vi "_PC_Pub lockPrompt.vi"(0 "Enable":bool=TRUE, 5 "error in (no error)":errorcluster) -> (17 "New Group Name":string, 18 "OK":bool, 19 "error out":errorcluster)   [LabVIEW 2018]
doc: "Displays a standard dialog box that prompts users to enter information, such as a user name and password.\n--------------------\n\nThis Express VI is configured as follows:\n\nMessage to Display to the User:Add Group Name?\nThe inputs are: \nText Entry Box: New Group Name"
panel:
  in  "New Group Name":string
  out "String":string="Add Group Name?"
  in  "Cancel":bool
  in  "OK2":bool
  in  "OK1":bool
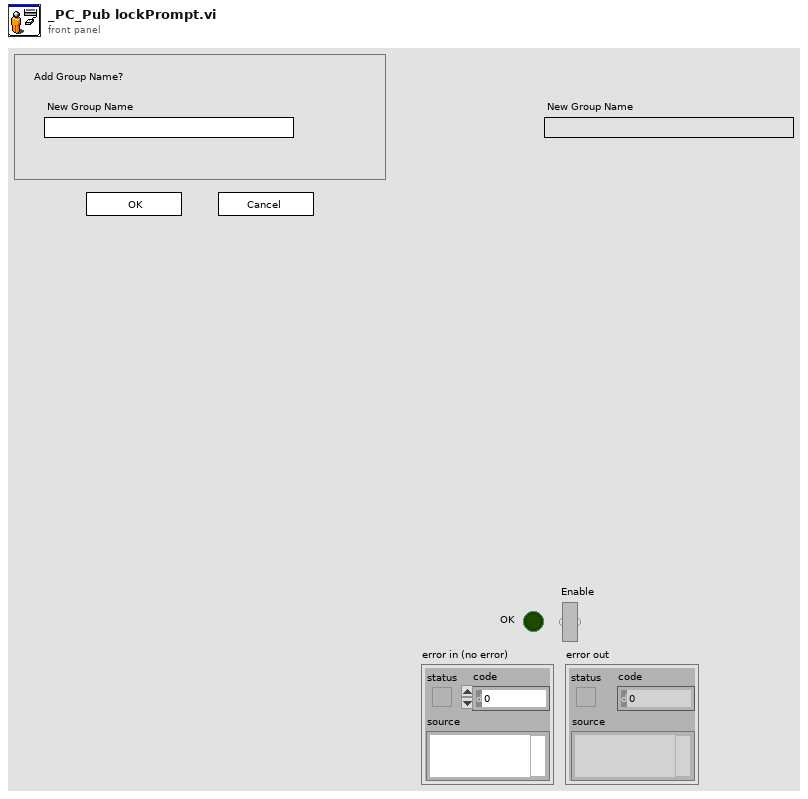
[diagram p1: front panel]
types:
  T1 = cluster{"Input Name":string, "Input Data Type":i32}[]
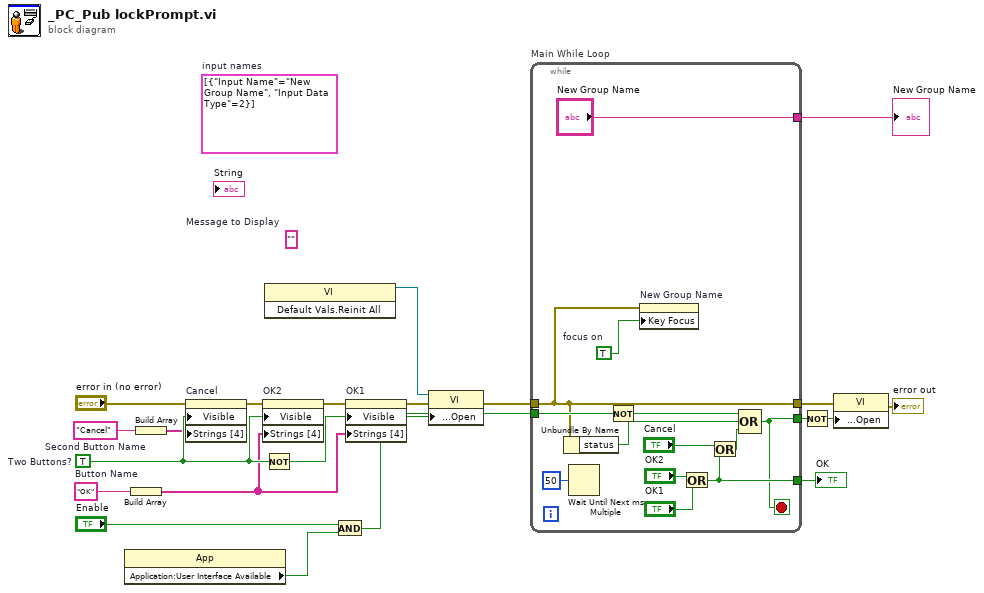
[diagram p0: block diagram]
diagram:
  (unwired) T1 [{"Input Name"="New Group Name", "Input Data Type"=2}]  # input names
  w13 = "Cancel"  # Second Button Name
  w11 = "OK"  # Button Name
  (unwired) ""  # Message to Display
  w21 = TRUE  # Two Buttons?
  n1 = property class="App"() -> ("Application:User Interface Available"=w3:bool)  [unwired: 2 in, 2 out]
  n2 = Build Array(w11) -> (w12:string[])
  n3 = Build Array(w13) -> (w14:string[])
  n4 = property on="Cancel" class="Bool"(error in="error in (no error)", "Visible"=w21, "Strings [4]"=w14) -> (error out=w18:errorcluster)  [unwired: 1 in, 1 out]
  n5 = property on="OK2" class="Bool"(error in=w18, "Visible"=w21, "Strings [4]"=w12) -> (error out=w17:errorcluster)  [unwired: 1 in, 1 out]
  n6 = Not(x=w21) -> (.not. x?=w19:bool)
  n7 = invoke class="VI" method="Default Vals.Reinit All"() -> (reference out=w2:refnum<vi>)  [unwired: 3 in, 2 out]
  n8 = And(x="Enable", y=w3) -> (x .and. y?=w4:bool)
  n9 = property on="OK1" class="Bool"(error in=w17, "Visible"=w19, "Strings [4]"=w12) -> (error out=w10:errorcluster)  [unwired: 1 in, 1 out]
  n10 = property class="VI"(reference=w2, error in=w10, "Front Panel Window:Open"=w4) -> (error out=w9:errorcluster)  [unwired: 1 out]
  n11 = while "Main While Loop" {
    tunnel: [w31] -> w20
    tunnel: w4 -> [w29]
    tunnel: [w27] -> w15
    tunnel: w9 -> [w23]
    tunnel: [w23] -> w7
    tunnel: ["New Group Name"] -> w1
    stop <- w27 stop-if-true
    w22 = TRUE  # focus on
    n12 = Unbundle By Name(w23) -> ("status"=w25:bool)
    n13 = Wait Until Next ms Multiple(millisecond multiple=u32 50) -> ()  [unwired: 1 out]
    n14 = Not(x=w29) -> (.not. x?=w28:bool)
    n15 = property on="New Group Name" class="Str"(error in=w23, "Key Focus"=w22) -> ()  [unwired: 1 in, 2 out]
    n16 = Or(x="OK2", y="OK1") -> (x .or. y?=w31:bool)
    n17 = Or(x="Cancel", y=w31) -> (x .or. y?=w26:bool)
    n18 = Compound Arithmetic op=OR(w28, w25, w26) -> (w27:bool)
  }
  "OK" <- w20
  "New Group Name" <- w1
  n19 = Not(x=w15) -> (.not. x?=w16:bool)
  n20 = property class="VI"(error in=w7, "Front Panel Window:Open"=w16) -> (error out=→"error out":errorcluster)  [unwired: 1 in, 1 out]
